vi "hse-configuration_ReadDoubleKey.vi"(8 "error in (no error)":errorcluster, 9 "Key":string, 10 "Section":string, 11 "hse-config-ini in":refnum<class "hse-config-ini.lvclass">) -> (0 "error out":errorcluster, 2 "Value":dbl, 3 "hse-config-ini out":refnum<class "hse-config-ini.lvclass">)   [LabVIEW 2020, in "hse-config-ini.lvclass"]
doc: "Reads the numeric configuration value (I32) identified by <b>section</b> and <b>key</b> from the configuration object\n\n____\nHAMPEL SOFTWARE ENGINEERING v3.8.0 (2023-12-18 14:41)"
uses:
  hse-config-ini.lvclass
  hse-misc/hse-misc.lvlib
  hse-misc/Conversion/ConvertStringToFloat_Scalar.vi
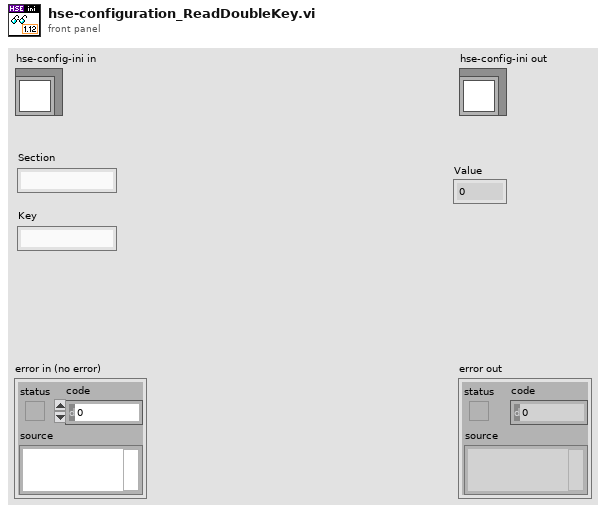
[diagram p1: front panel]
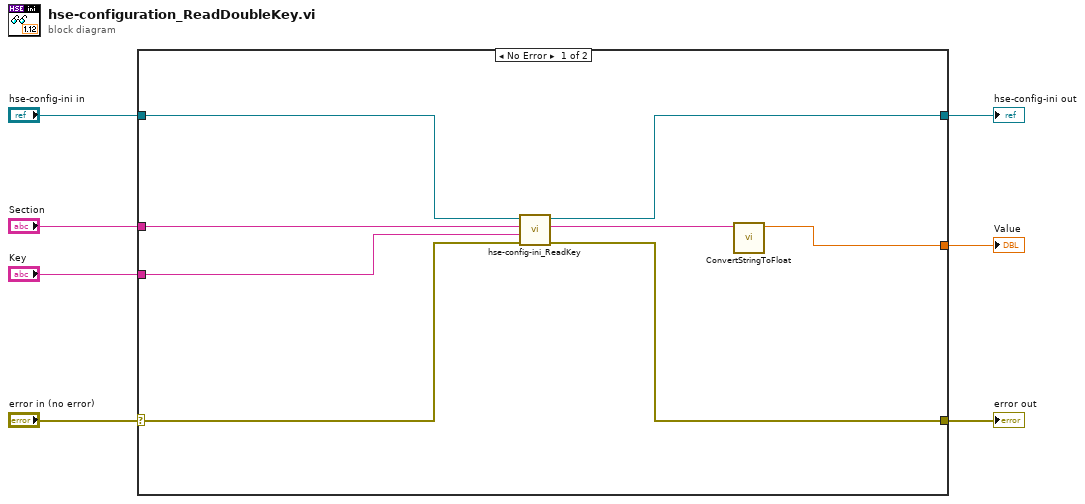
[diagram p0: block diagram]
diagram:
  n1 = case shown="No Error" "error in (no error)" {
    selector: "error in (no error)" -> [w11 w17]
    tunnel: [w10 w17] -> w7
    tunnel: "hse-config-ini in" -> [w15 w16]
    tunnel: [w14 w16] -> w4
    tunnel: "Section" -> [w13 _]
    tunnel: "Key" -> [w12 _]
    tunnel: [w8 _] -> w6
    frame No Error {
      n2 = call "hse-config-ini_ReadKey.vi"("error in (no error)"=w11, "Key"=w12, "Section"=w13, "hse-config-ini in"=w15) -> ("error out"=w10:errorcluster, "String"=w9:string, "hse-config-ini out"=w14:refnum<class "hse-config-ini.lvclass">)  [unwired: 5 in]
      n3 = call-poly "ConvertStringToFloat.vi"("String"=w9) -> ("Double"=w8:dbl)  [unwired: 9 in, 1 out]
    }
    frame Error {
    }
  }
  "error out" <- w7
  "hse-config-ini out" <- w4
  "Value" <- w6
